vi "main.vi"() -> ()   [LabVIEW 2015]
uses:
  controls/state.ctl
  controls/sprinkler data.ctl
  controls/timerstatus.ctl
panel:
  in  "error in (no error)":errorcluster
  out "error out":errorcluster
  in  "Simulation Controls":T1 {"Water Pressure Sensor (%)" scale=0.0..100.0}
  in  "Controls":T2
  in  "Zone Setup Array":cluster{"Zone Selector":string, "Timing":dbl}[](array[cluster])
  out "Controller Status":string
  out "Zone Indicators":T3
  # "Rain"
  # "No Rain"
  # "Continuous"
  # "Single"
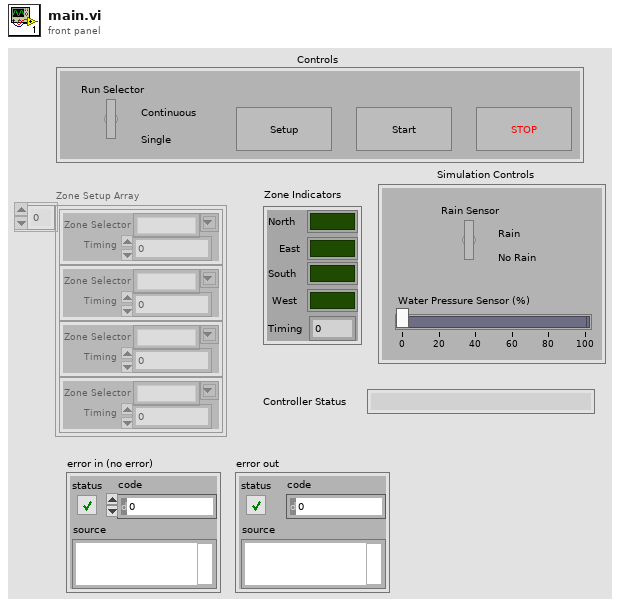
[diagram p1: front panel]
types:
  T1 = cluster{"Rain Sensor":bool, "Water Pressure Sensor (%)":dbl}
  T2 = cluster{"Run Selector":bool, "Setup":bool, "Start":bool, "Stop":bool}
  T3 = cluster{"North":bool, "East":bool, "South":bool, "West":bool, "Timing":u32}
  T4 = typedef "state.ctl" = enum16{"Error under range", "Exit", "Initialize", "Start", "Error", "Run", "Setup", "Low pressure", "Rain", "Idle"}
  T5 = enum8{"Enabled", "Disabled", "Disabled and Grayed Out"}
  T6 = typedef "timerstatus.ctl" = enum16{"Stop", "Start"}
  T7 = typedef "sprinkler data.ctl" = cluster{"Zone Setup Array":cluster{"Zone Selector":string, "Timing":dbl}[], "Zone Indicators":cluster{"North":bool, "East":bool, "South":bool, "West":bool, "Timing":u32}, "order":i32}
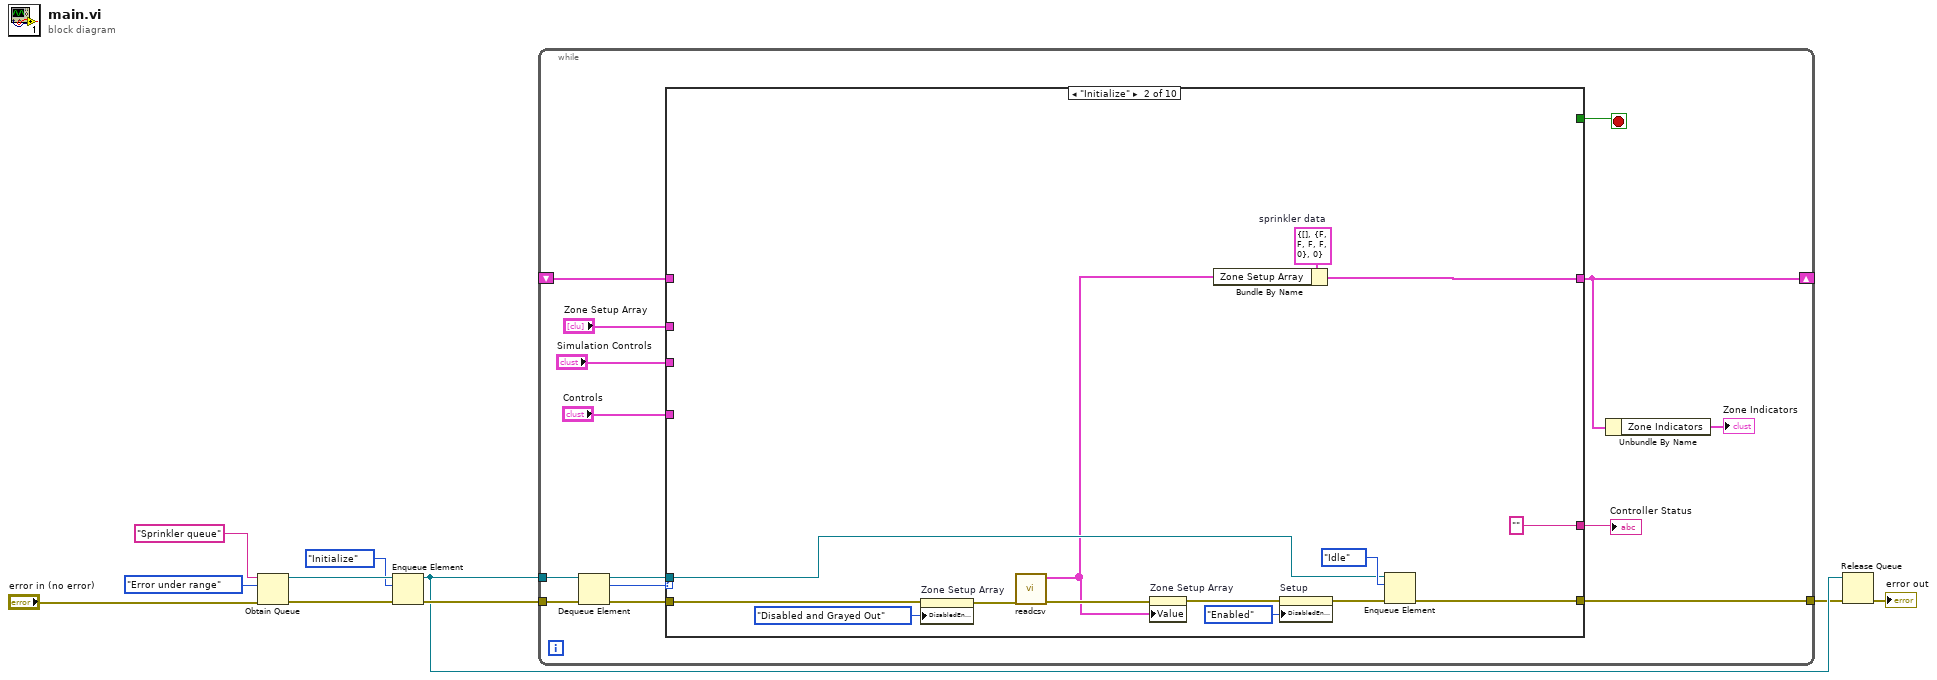
[diagram p0: block diagram]
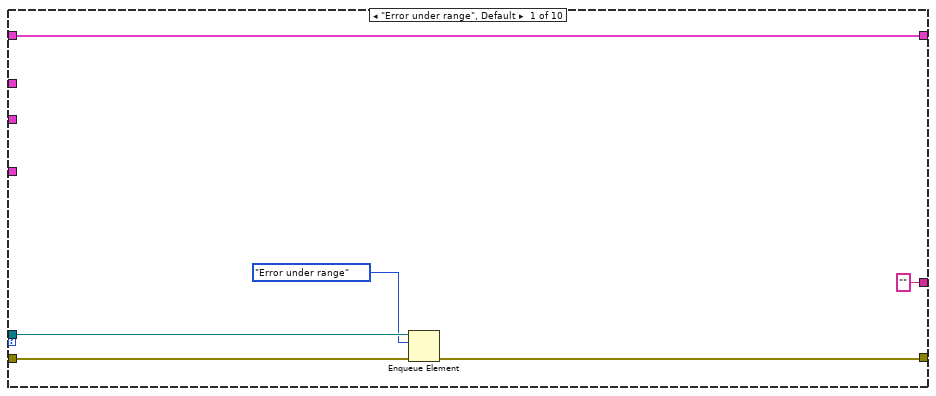
[diagram p2: hidden frame]
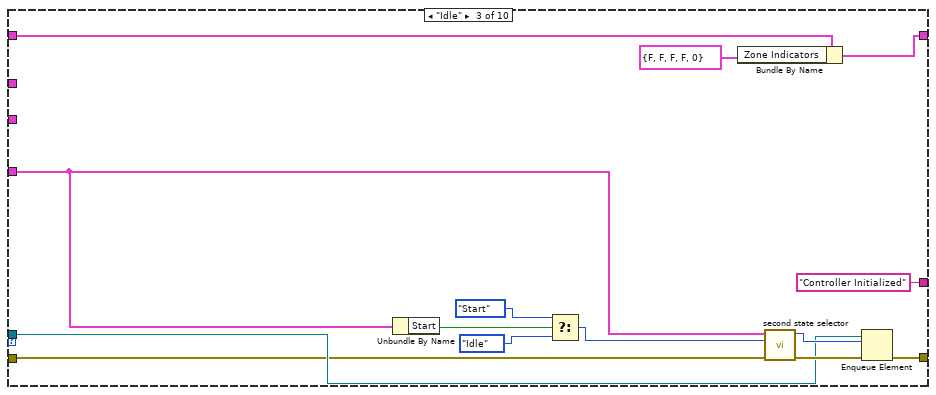
[diagram p3: hidden frame]
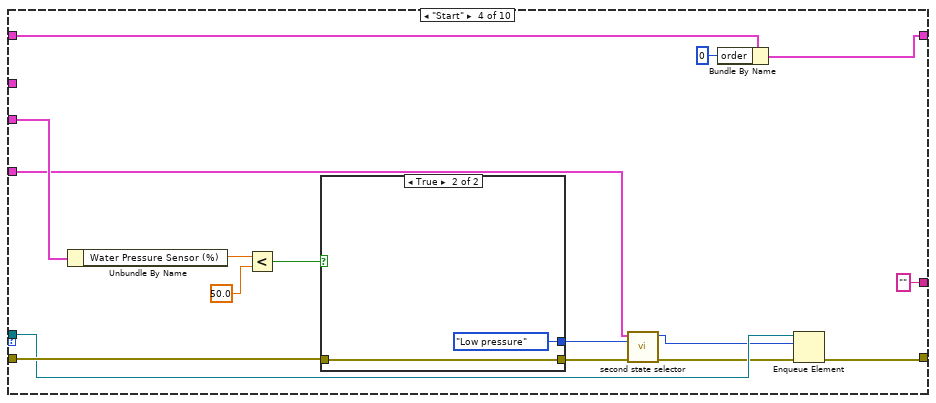
[diagram p4: hidden frame]
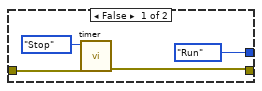
[diagram p5: hidden frame]
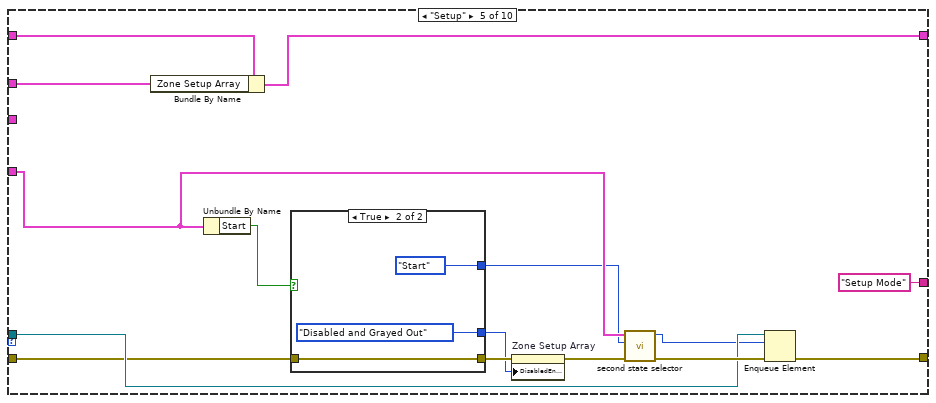
[diagram p6: hidden frame]
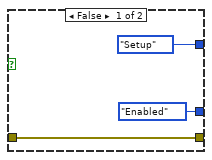
[diagram p7: hidden frame]
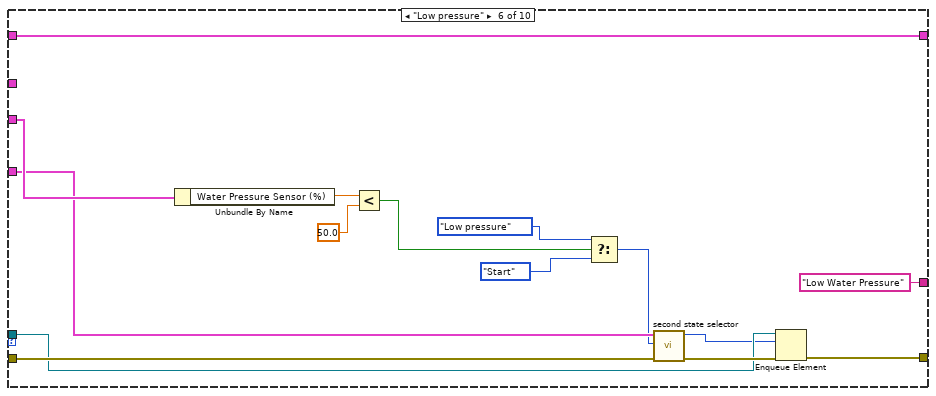
[diagram p8: hidden frame]
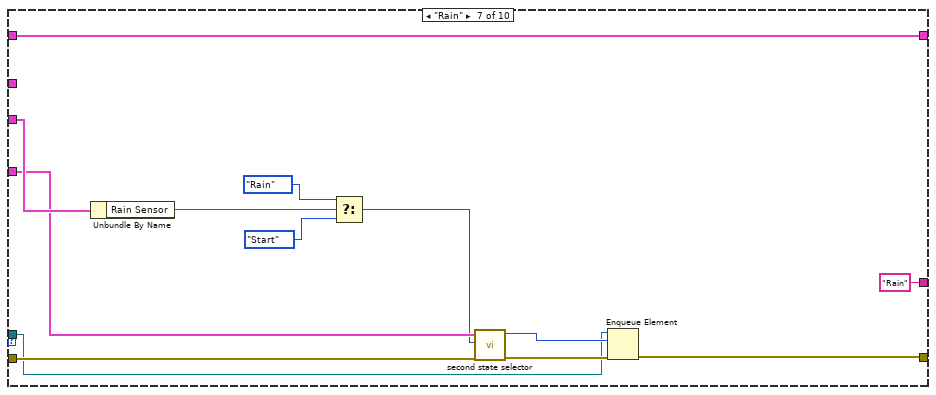
[diagram p9: hidden frame]
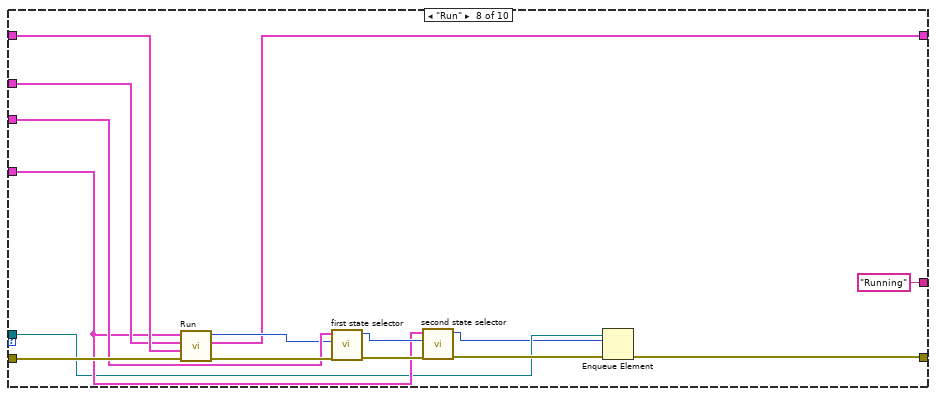
[diagram p10: hidden frame]
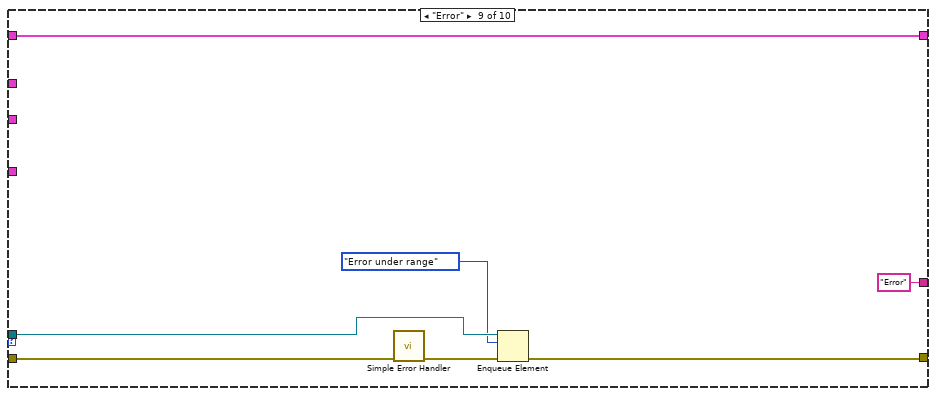
[diagram p11: hidden frame]
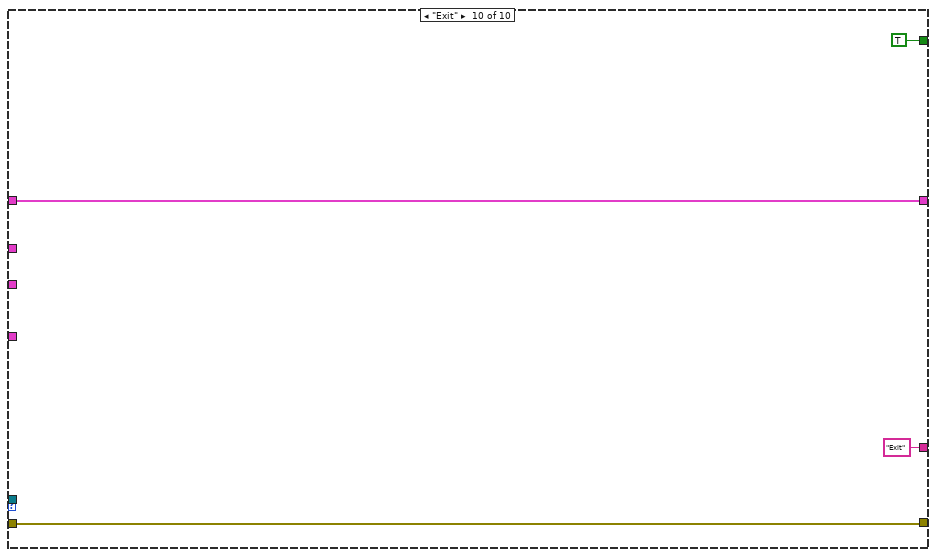
[diagram p12: hidden frame]
diagram:
  n1 = Obtain Queue(name (unnamed)="Sprinkler queue", element data type=state."Error under range" ("state"), error in (no error)="error in (no error)") -> (queue out=w8:refnum<queue>, error out=w10:errorcluster)  [unwired: 2 in, 1 out]
  n2 = Enqueue Element(queue=w8, element=state."Initialize", error in (no error)=w10) -> (queue out=w4:refnum<queue>, error out=w9:errorcluster)  [unwired: 1 in, 1 out]
  n3 = while {
    tunnel: w9 -> [w24]
    tunnel: w4 -> [w23]
    tunnel: [w18] -> w3
    shift-right: [w12] -> _
    shift-left: _ -> [w14]
    stop <- w15 stop-if-true
    n4 = Dequeue Element(queue=w23, error in (no error)=w24) -> (queue out=w20:refnum<queue>, element=w22:T4, error out=w21:errorcluster)  [unwired: 1 in, 1 out]
    n5 = case shown="\"Initialize\"" w22 {
      tunnel: w21 -> [w28 w39 w52 w74 w86 w107 w127 w144 w151 w155]
      tunnel: w20 -> [w26 w40 w54 w66 w89 w103 w118 w132 w147 _]
      tunnel: "Zone Setup Array" -> [_ _ _ _ w93 _ _ w142 _ _]
      tunnel: [w27 w42 w56 w63 w91 w109 w117 w133 w145 w155] -> w18
      tunnel: "Controls" -> [_ _ w58 w67 w87 w105 w124 w135 _ _]
      tunnel: "Simulation Controls" -> [_ _ _ w73 _ w114 w126 w140 _ _]
      tunnel: [_ _ _ _ _ _ _ _ _ TRUE] -> w15
      tunnel: [w30 w34 w46 w59 w92 w108 w128 w138 w150 w153] -> w12
      tunnel: w14 -> [w30 _ w47 w61 w94 w108 w128 w143 w150 w153]
      tunnel: ["" "" "Controller Initialized" "" "Setup Mode" "Low Water Pressure" "Rain" "Running" "Error" "Exit"] -> w13
      frame "Error under range", Default {
        n6 = Enqueue Element(queue=w26, element=state."Error under range", error in (no error)=w28) -> (error out=w27:errorcluster)  [unwired: 1 in, 2 out]
      }
      frame "Initialize" {
        w36 = T7 {"Zone Setup Array"=[], "Zone Indicators"={"North"=FALSE, "East"=FALSE, "South"=FALSE, "West"=FALSE, "Timing"=0}, "order"=0}  # sprinkler data
        n7 = property on="Zone Setup Array" class="Arr (strict)"(error in=w39, "DisabledEnum"=T5."Disabled and Grayed Out" ("Disabled")) -> (error out=w38:errorcluster)  [unwired: 1 in, 1 out]
        n8 = call "readcsv.vi"("error in"=w38) -> ("error out"=w44:errorcluster, "Zone Setup Array"=w35:cluster{"Zone Selector":string, "Timing":dbl}[])  [unwired: 9 in]
        n9 = property on="Zone Setup Array" class="Arr (strict)"(error in=w44, "Value"=w35) -> (error out=w33:errorcluster)  [unwired: 1 in, 1 out]
        n10 = Bundle By Name(cluster=w36, "Zone Setup Array"=w35) -> (w34:T7)
        n11 = property on="Setup" class="Bool"(error in=w33, "DisabledEnum"=T5."Enabled" ("Disabled")) -> (error out=w32:errorcluster)  [unwired: 1 in, 1 out]
        n12 = Enqueue Element(queue=w40, element=state."Idle", error in (no error)=w32) -> (error out=w42:errorcluster)  [unwired: 1 in, 2 out]
      }
      frame "Idle" {
        n13 = Unbundle By Name(w58) -> ("Start"=w51:bool)
        n14 = Select(t=state."Start" ("element"), s=w51, f=state."Idle" ("element")) -> (s? t:f=w48:T4)
        n15 = Bundle By Name(cluster=w47, "Zone Indicators"=T3 {"North"=FALSE, "East"=FALSE, "South"=FALSE, "West"=FALSE, "Timing"=0}) -> (w46:T7)
        n16 = call "second state selector.vi"("error in"=w52, "state"=w48, "Controls"=w58) -> ("error out"=w57:errorcluster, "state out"=w55:T4)  [unwired: 7 in]
        n17 = Enqueue Element(queue=w54, element=w55, error in (no error)=w57) -> (error out=w56:errorcluster)  [unwired: 1 in, 2 out]
      }
      frame "Start" {
        n18 = Unbundle By Name(w73) -> ("Water Pressure Sensor (%)"=w72:dbl)
        n19 = Less?(x=w72, y=50.0) -> (x < y?=w70:bool)
        n20 = case shown="True" w70 {
          tunnel: [w77 w80] -> w69
          tunnel: w74 -> [w78 w80]
          tunnel: [state."Run" ("element") state."Low pressure" ("element")] -> w68
          frame False {
            n21 = call "timer.vi"("error in"=w78, "timerstat"=timerstatus."Stop") -> ("error out"=w77:errorcluster)  [unwired: 7 in, 2 out]
          }
          frame True {
          }
        }
        n22 = call "second state selector.vi"("error in"=w69, "state"=w68, "Controls"=w67) -> ("error out"=w64:errorcluster, "state out"=w65:T4)  [unwired: 7 in]
        n23 = Bundle By Name(cluster=w61, "order"=0) -> (w59:T7)
        n24 = Enqueue Element(queue=w66, element=w65, error in (no error)=w64) -> (error out=w63:errorcluster)  [unwired: 1 in, 2 out]
      }
      frame "Setup" {
        n25 = Bundle By Name(cluster=w94, "Zone Setup Array"=w93) -> (w92:T7)
        n26 = Unbundle By Name(w87) -> ("Start"=w82:bool)
        n27 = case shown="True" w82 {
          tunnel: w86 -> [w96 w101]
          tunnel: [w96 w101] -> w85
          tunnel: [state."Setup" ("element") state."Start" ("element")] -> w84
          tunnel: [T5."Enabled" ("Disabled") T5."Disabled and Grayed Out" ("Disabled")] -> w81
          frame False {
          }
          frame True {
          }
        }
        n28 = property on="Zone Setup Array" class="Arr (strict)"(error in=w85, "DisabledEnum"=w81) -> (error out=w83:errorcluster)  [unwired: 1 in, 1 out]
        n29 = call "second state selector.vi"("error in"=w83, "state"=w84, "Controls"=w87) -> ("error out"=w90:errorcluster, "state out"=w88:T4)  [unwired: 7 in]
        n30 = Enqueue Element(queue=w89, element=w88, error in (no error)=w90) -> (error out=w91:errorcluster)  [unwired: 1 in, 2 out]
      }
      frame "Low pressure" {
        n31 = Unbundle By Name(w114) -> ("Water Pressure Sensor (%)"=w116:dbl)
        n32 = Less?(x=w116, y=50.0) -> (x < y?=w112:bool)
        n33 = Select(t=state."Low pressure" ("element"), s=w112, f=state."Start" ("element")) -> (s? t:f=w104:T4)
        n34 = call "second state selector.vi"("error in"=w107, "state"=w104, "Controls"=w105) -> ("error out"=w106:errorcluster, "state out"=w102:T4)  [unwired: 7 in]
        n35 = Enqueue Element(queue=w103, element=w102, error in (no error)=w106) -> (error out=w109:errorcluster)  [unwired: 1 in, 2 out]
      }
      frame "Rain" {
        n36 = Unbundle By Name(w126) -> ("Rain Sensor"=w125:bool)
        n37 = Select(t=state."Rain" ("element"), s=w125, f=state."Start" ("element")) -> (s? t:f=w121:T4)
        n38 = call "second state selector.vi"("error in"=w127, "state"=w121, "Controls"=w124) -> ("error out"=w120:errorcluster, "state out"=w119:T4)  [unwired: 7 in]
        n39 = Enqueue Element(queue=w118, element=w119, error in (no error)=w120) -> (error out=w117:errorcluster)  [unwired: 1 in, 2 out]
      }
      frame "Run" {
        n40 = call "Run.vi"("error in (no error)"=w144, "sprinkler data in"=w143, "Zone Setup Array"=w142, "Controls"=w135) -> ("error out"=w141:errorcluster, "sprinkler data out"=w138:T7, "state"=w139:T4)  [unwired: 5 in]
        n41 = call "first state selector.vi"("error in"=w141, "state"=w139, "Simulation Controls"=w140) -> ("error out"=w137:errorcluster, "state out"=w136:T4)  [unwired: 7 in]
        n42 = call "second state selector.vi"("error in"=w137, "state"=w136, "Controls"=w135) -> ("error out"=w134:errorcluster, "state out"=w131:T4)  [unwired: 7 in]
        n43 = Enqueue Element(queue=w132, element=w131, error in (no error)=w134) -> (error out=w133:errorcluster)  [unwired: 1 in, 2 out]
      }
      frame "Error" {
        n44 = call <vilib>:"Simple Error Handler.vi"("error in (no error)"=w151) -> ("error out"=w148:errorcluster)  [unwired: 4 in, 4 out]
        n45 = Enqueue Element(queue=w147, element=state."Error under range", error in (no error)=w148) -> (error out=w145:errorcluster)  [unwired: 1 in, 2 out]
      }
      frame "Exit" {
      }
    }
    "Controller Status" <- w13
    n46 = Unbundle By Name(w12) -> ("Zone Indicators"=→"Zone Indicators":T3)
  }
  n47 = Release Queue(queue=w4, error in (no error)=w3) -> (error out=→"error out":errorcluster)  [unwired: 1 in, 2 out]
